vi "1 SiO2 Material Properties.vi"(6 "NS Base Area":dbl, 8 "Silicon DiOxide Thickness  in":dbl, 9 "m-nm SiO2 in":dbl, 11 "Energy (Heat; I^2R)":dbl) -> (1 "SiO2 Specfic Heat Capacity":dbl, 2 "Mass SiO2":dbl, 3 "SilO2 Density":dbl, 4 "Delta Temp Change SiO2":dbl, 5 "Volume SiO2":dbl, 7 "Sio2 Thickness":dbl)   [LabVIEW 2020]
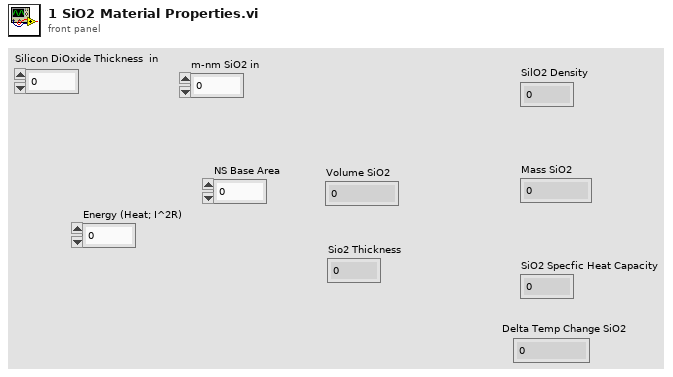
[diagram p1: front panel]
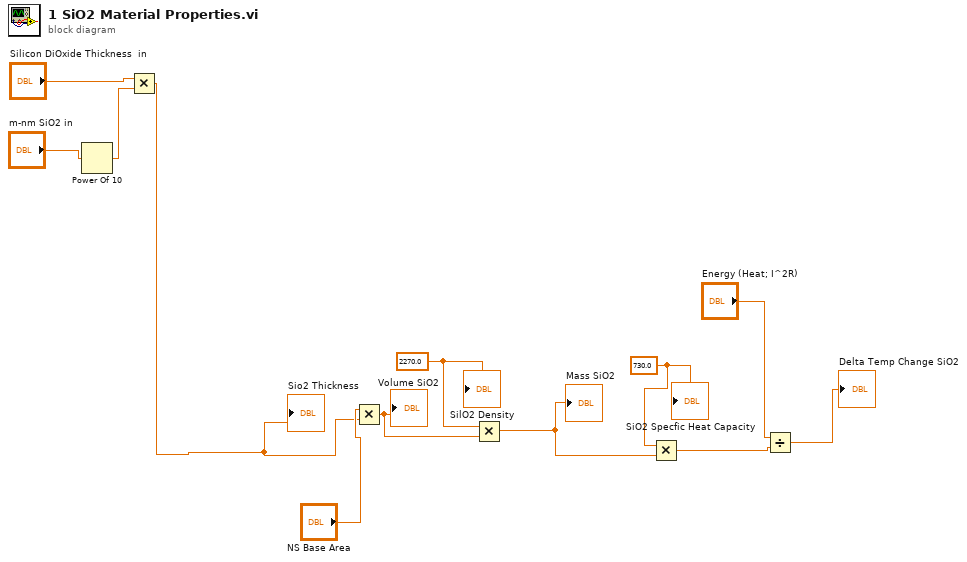
[diagram p0: block diagram]
diagram:
  w7 = 730.0 ("Silicon Specfic Heat Capacity 2")
  w5 = 2270.0 ("Silicon Dioxide Density 2")
  n1 = Power Of 10(x="m-nm SiO2 in") -> (10^x=w2:dbl)
  n2 = Multiply(x="Silicon DiOxide Thickness  in", y=w2) -> (x*y=w1:dbl)
  "Sio2 Thickness" <- w1
  n3 = Multiply(x="NS Base Area", y=w1) -> (x*y=w6:dbl)
  "Volume SiO2" <- w6
  n4 = Multiply(x=w5, y=w6) -> (x*y=w8:dbl)
  "Mass SiO2" <- w8
  n5 = Multiply(x=w7, y=w8) -> (x*y=w10:dbl)
  n6 = Divide(x="Energy (Heat; I^2R)", y=w10) -> (x/y=→"Delta Temp Change SiO2":dbl)
  "SilO2 Density" <- w5
  "SiO2 Specfic Heat Capacity" <- w7
